vi "Shell Execute.vi"(7 "wait until completion?":bool=TRUE, 8 "error in":errorcluster, 9 "arguments":string, 10 "target":string, 11 "working directory":string) -> (0 "error out":errorcluster, 1 "standard error":string, 2 "return code":i32, 3 "standard output":string)   [LabVIEW 2015]
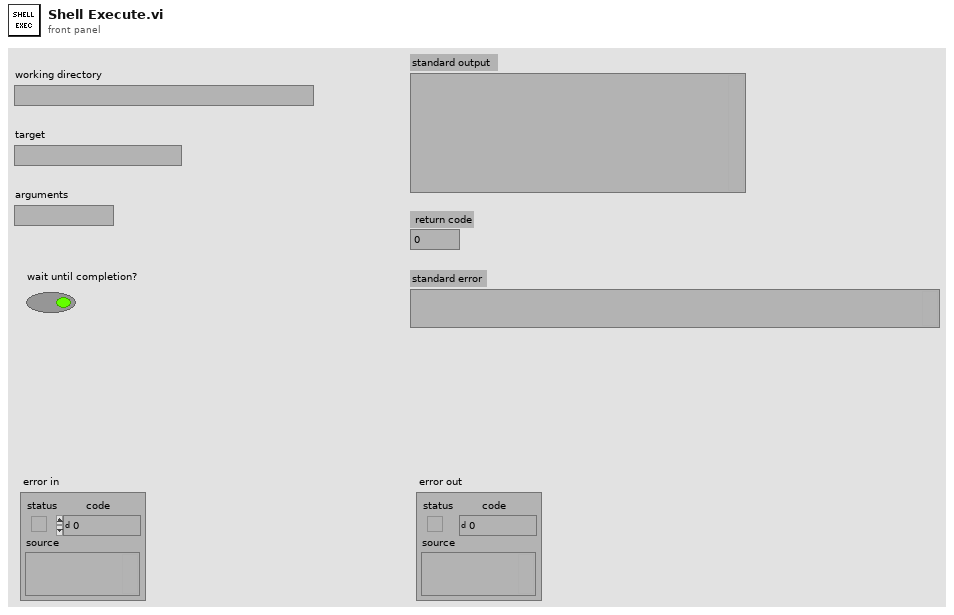
[diagram p1: front panel]
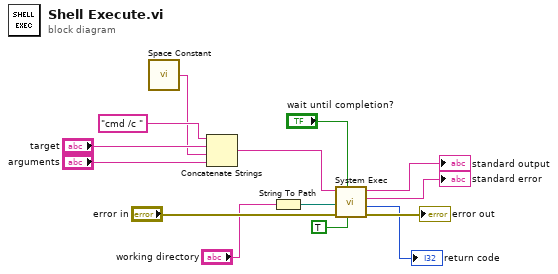
[diagram p0: block diagram]
diagram:
  n1 = call <vilib>:"Space Constant.vi"() -> ("String"=w6:string)
  n2 = Concatenate Strings("cmd /c " ("command line"), "target", w6, "arguments") -> (w4:string)
  n3 = String To Path(string="working directory") -> (path=w3:path)
  n4 = call <vilib>:"System Exec.vi"("run minimized? (F)"=TRUE, "wait until completion? (T)"="wait until completion?", "error in (no error)"="error in", "working directory"=w3, "command line"=w4) -> ("error out"=→"error out":errorcluster, "return code"=→"return code":i32, "standard error"=→"standard error":string, "standard output"=→"standard output":string)  [unwired: 3 in]
